vi "CMWexitALLTypes.vi"(8 "error in (no error)":errorcluster, 10 "Data Type":string, 11 "URL":string="VAC.VGHA_41677/PR") -> (0 "error out":errorcluster, 3 "CMWout":refnum<class "CMWSubscribe.lvclass">)   [LabVIEW 2014]
uses:
  <userlib>/_RADE/RIO/CMW/classes/CMWSubscribe/CMWSubscribe.lvclass
  <userlib>/_RADE/RIO/CMW/classes/CMWSubscribe/openCMWSubscribe.vi
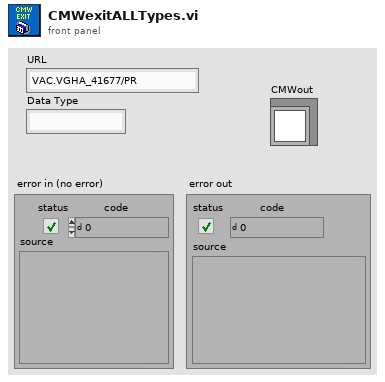
[diagram p1: front panel]
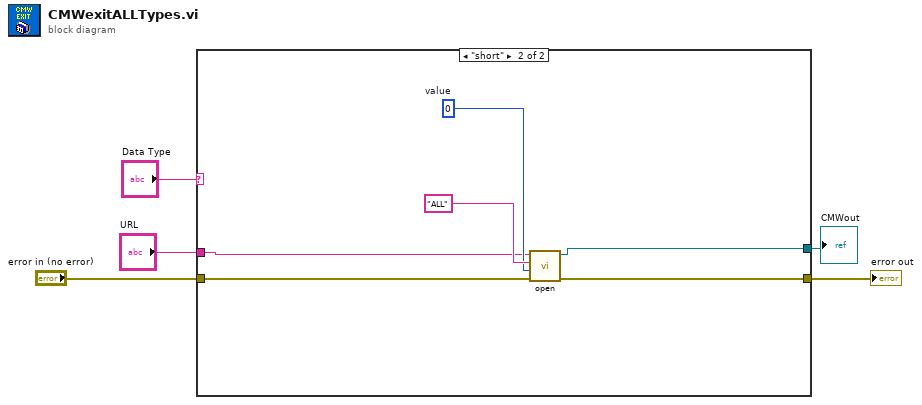
[diagram p0: block diagram]
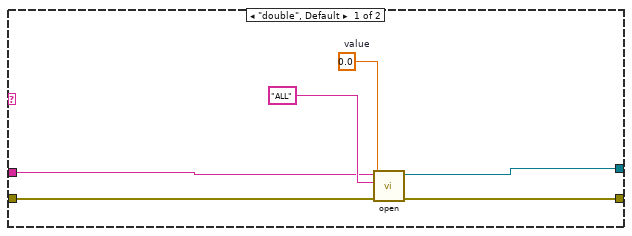
[diagram p2: hidden frame]
diagram:
  n1 = case shown="\"short\"" "Data Type" {
    tunnel: "error in (no error)" -> [w9 w16]
    tunnel: [w8 w15] -> w4
    tunnel: "URL" -> [w10 w13]
    tunnel: [w7 w12] -> w1
    frame "double", Default {
      w6 = sgl 0.0  # value
      n2 = call-poly <userlib>:"open.vi"("error in (no error)"=w9, "Data type"=w6, "Cycle"="ALL", "URL"=w10) -> ("error out"=w8:errorcluster, "Object out"=w7:refnum<class "CMWSubscribe.lvclass">)  [unwired: 6 in]
    }
    frame "short" {
      w14 = i16 0  # value
      n3 = call-poly <userlib>:"open.vi"("error in (no error)"=w16, "Data type"=w14, "Cycle"="ALL", "URL"=w13) -> ("error out"=w15:errorcluster, "Object out"=w12:refnum<class "CMWSubscribe.lvclass">)  [unwired: 6 in]
    }
  }
  "error out" <- w4
  "CMWout" <- w1
